vi "Initialize.vi"(8 "error in (no error)":errorcluster, 11 "CD Parameter Manager in":refnum<class "CD Parameter Manager.lvclass">) -> (0 "error out":errorcluster, 3 "CD Parameter Manager out":refnum<class "CD Parameter Manager.lvclass">)   [LabVIEW 2019, in "CD Parameter Manager API.lvlib" / "CD Parameter Manager.lvclass"]
uses:
  CD Parameter Manager.lvclass
  Double Parameter Class/Double Parameter.lvclass
  C:/Repositories/UI-Control-Initializer-API/Source/Parameter Class/Parameter.lvclass
  I32 Parameter Class/I32 Parameter.lvclass
  Boolean Parameter Class/Boolean Parameter.lvclass
  Parameter Class/Parameter.lvclass/Parameter.ctl
  CD Parameter Manager.lvclass/CD Parameter Manager.ctl
  Parameter Class/Member Accessors/Write Control label.vi
  Parameter Class/Parameter.lvclass
panel:
  in  "Control Properties":T1(array[cluster])
  in  "VI Refnum":refnum<vi>
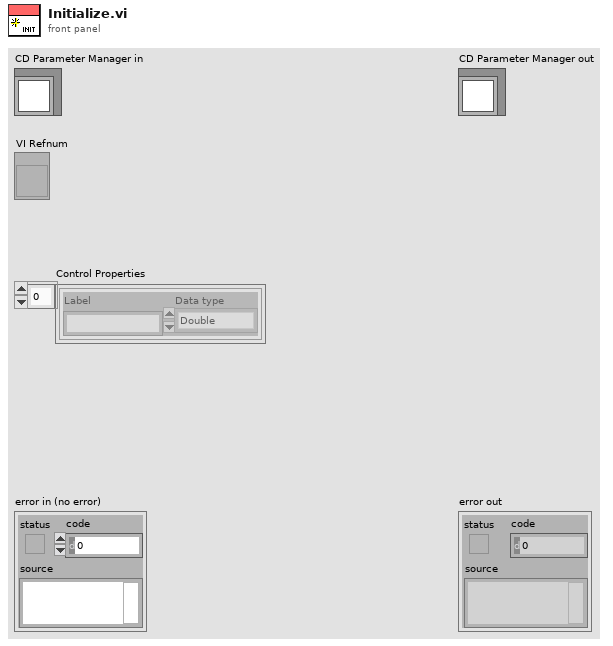
[diagram p1: front panel]
types:
  T1 = cluster{"Label":string, "Data type":enum16{"Double", "I32", "Boolean", "String"}}[]
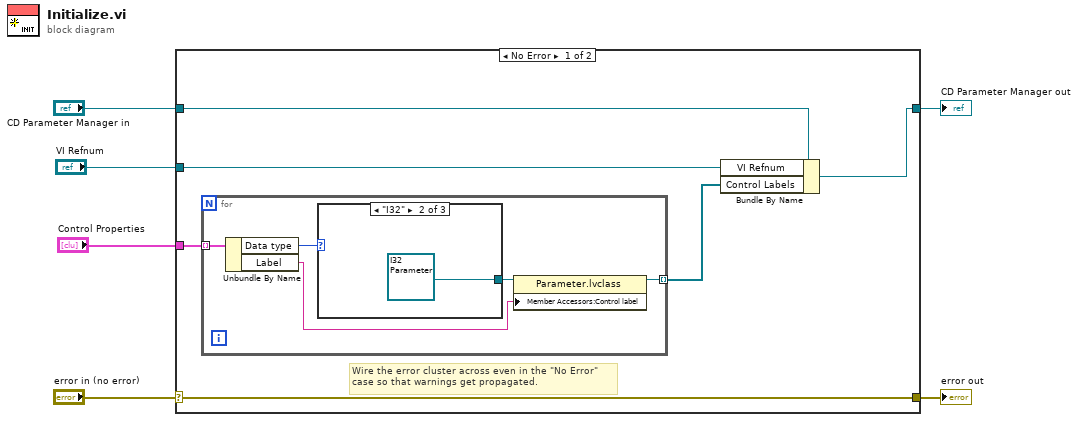
[diagram p0: block diagram]
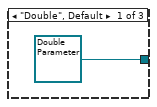
[diagram p2: hidden frame]
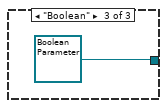
[diagram p3: hidden frame]
diagram:
  n1 = case shown="No Error" "error in (no error)" {
    selector: "error in (no error)" -> [w12 w22]
    tunnel: [w12 w22] -> w5
    tunnel: [w9 w21] -> w3
    tunnel: "CD Parameter Manager in" -> [w11 w21]
    tunnel: "VI Refnum" -> [w10 _]
    tunnel: "Control Properties" -> [w8 _]
    frame No Error {
      # "Wire the error cluster across even in the \"No Error\"\ncase so that warnings get propagated."
      n2 = for {
        tunnel: w8 -> [w17] mode=indexing
        tunnel: [w14] -> w7 mode=indexing
        n3 = Unbundle By Name(w17) -> ("Data type"=w16:enum16{"Double", "I32", "Boolean", "String"}, "Label"=w13:string)
        n4 = case shown="\"I32\"" w16 {
          tunnel: [refnum<class "Double Parameter.lvclass"> refnum ("CD Parameter Manager API.lvlib:Double Parameter.lvclass") refnum<class "I32 Parameter.lvclass"> refnum ("CD Parameter Manager API.lvlib:I32 Parameter.lvclass") refnum<class "Boolean Parameter.lvclass"> refnum ("CD Parameter Manager API.lvlib:Boolean Parameter.lvclass")] -> w15
          frame "Double", Default {
          }
          frame "I32" {
          }
          frame "Boolean" {
          }
        }
        n5 = property class="Parameter.lvclass"(reference=w15, "Member Accessors:Control label"=w13) -> (reference out=w14:refnum<class "Parameter.lvclass">)  [unwired: 1 in, 1 out]
      }
      n6 = Bundle By Name(cluster=w11, "VI Refnum"=w10, "Control Labels"=w7) -> (w9:refnum<class "CD Parameter Manager.lvclass">)
    }
    frame Error {
    }
  }
  "error out" <- w5
  "CD Parameter Manager out" <- w3
